vi "Query Active DUT SIM Slot Catalog.vi"(8 "error in (no error)":errorcluster, 11 "VISA resource name":refnum<visa-resource-name>) -> (0 "error out":errorcluster, 2 "SIM Slots":string, 3 "VISA resource name out":refnum<visa-resource-name>)   [LabVIEW 2020, in "Rohde&Schwarz CMXP Base.lvlib"]
doc: "Queries all SIM slots of the active DUT. For each SIM slot, the slot number and the name of the referenced profile are returned: {<SimSlotNo>, <SimProfileName>}1, {...}2, ...\n\nAttribute:\nRSCMXPBASE_ATTR_ACTIVE_DUT_SIM_SLOT_CATALOG\n\nRemote-control command:\nCATalog:DUT:SIMSlot?"
uses:
  <instrlib>/Rohde&Schwarz CMXP Base/Rohde&Schwarz CMXP Base.lvlib
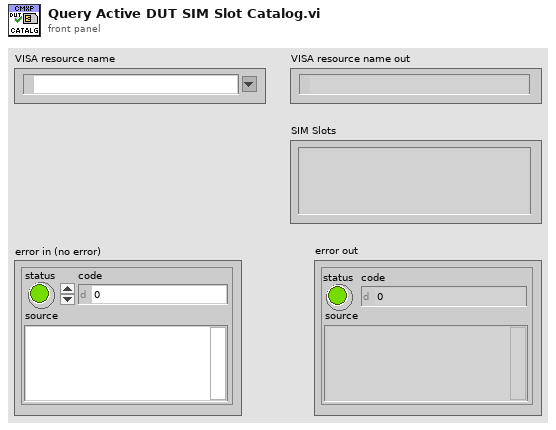
[diagram p1: front panel]
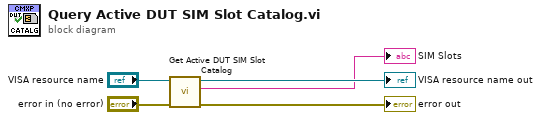
[diagram p0: block diagram]
diagram:
  n1 = call "Get Active DUT SIM Slot Catalog"("error in (no error)"="error in (no error)", "instrument handle"="VISA resource name") -> ("error out"=→"error out":errorcluster, "Active DUT SIM Slot Catalog"=→"SIM Slots":string, "instrument handle out"=→"VISA resource name out":refnum<visa-resource-name>)  [unwired: 7 in]
